vi "Full Adder.vi"(2 "c in":bool, 3 "b":bool, 4 "a":bool) -> (0 "c out":bool, 1 "s":bool)   [LabVIEW 2012]
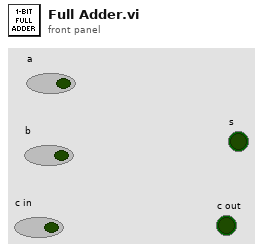
[diagram p1: front panel]
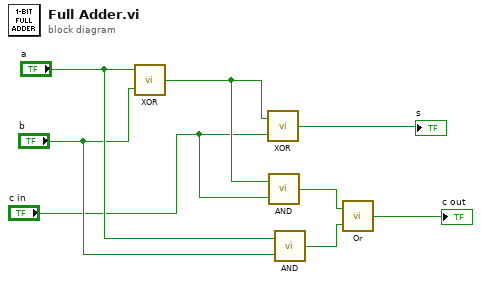
[diagram p0: block diagram]
diagram:
  n1 = call "XOR.vi"("b"="b", "a"="a") -> ("x"=w3:bool)
  n2 = call "XOR.vi"("b"="c in", "a"=w3) -> ("x"=→"s":bool)
  n3 = call "AND.vi"("b"="c in", "a"=w3) -> ("x"=w7:bool)
  n4 = call "AND.vi"("b"="b", "a"="a") -> ("x"=w6:bool)
  n5 = call "Or.vi"("b"=w6, "a"=w7) -> ("x"=→"c out":bool)
